vi "Station Initialize.vi"(8 "error in (no error)":errorcluster, 11 "Station in":refnum<class "Station.lvclass">) -> (0 "error out":errorcluster, 2 "All Passed?":bool, 3 "Station out":refnum<class "Station.lvclass">)   [LabVIEW 2018, in "Station.lvclass"]
uses:
  Station.lvclass
  Station Support/Controls/Server Control.ctl
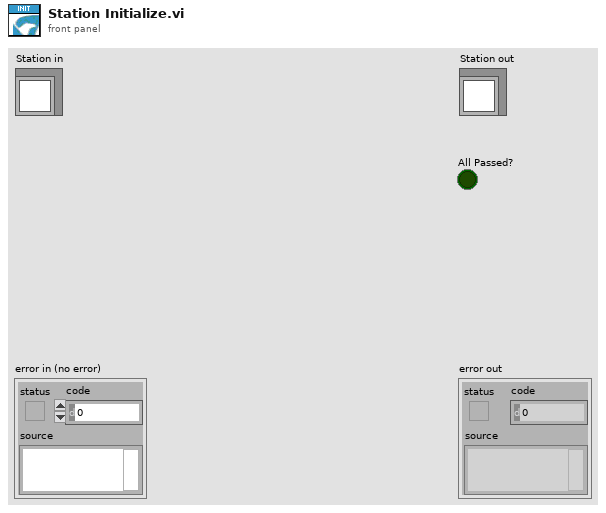
[diagram p1: front panel]
types:
  T1 = typedef "Server Control.ctl" = enum16{"Open New Reference", "Remove Reference", "Kill Server", "Set Station Ref", "Get Station Ref"}
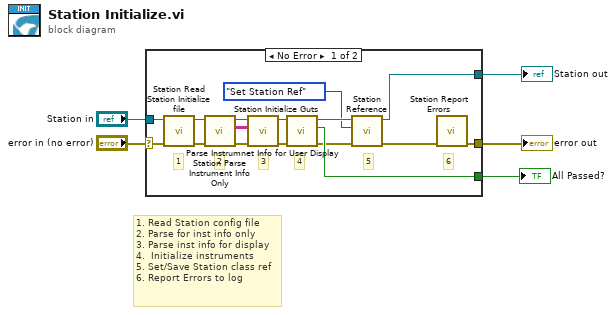
[diagram p0: block diagram]
diagram:
  # "1. Read Station config file\n2. Parse for inst info only\n3. Parse inst info for display\n4.  Initialize instruments\n5. Set/Save Station class ref\n6. Report Errors to log"
  n1 = case shown="No Error" "error in (no error)" {
    selector: "error in (no error)" -> [w21 w23]
    tunnel: [w11 w23] -> w4
    tunnel: [w8 w22] -> w2
    tunnel: "Station in" -> [w20 w22]
    tunnel: [w12 _] -> w1
    frame No Error {
      # "6"
      # "5"
      # "4"
      # "3"
      # "2"
      # "1"
      n2 = call "Station Read Station Initialize file.vi"("error in (no error)"=w21, "Station in"=w20) -> ("error out"=w19:errorcluster, "Station out"=w18:refnum<class "Station.lvclass">)  [unwired: 8 in]
      n3 = call "Station Parse Instrument Info Only.vi"("error in (no error)"=w19, "Station in"=w18) -> ("error out"=w17:errorcluster, "Inst Info only output"=w15:string[][], "Station out"=w16:refnum<class "Station.lvclass">)  [unwired: 7 in]
      n4 = call "Parse Instrumnet Info for User Display.vi"("error in (no error)"=w17, "Inst Info only output"=w15, "Station in"=w16) -> ("error out"=w13:errorcluster, "Station out"=w14:refnum<class "Station.lvclass">)  [unwired: 7 in]
      n5 = call "Station Initialize Guts.vi"("error in (no error)"=w13, "Station in"=w14) -> ("error out"=w10:errorcluster, "All Passed?"=w12:bool, "Station out"=w9:refnum<class "Station.lvclass">)  [unwired: 7 in]
      n6 = call "Station Reference.vi"("error in (no error)"=w10, "Action (0: Create)"=Server_Control."Set Station Ref", "Station in"=w9) -> ("error out"=w7:errorcluster, "Station out"=w8:refnum<class "Station.lvclass">)  [unwired: 7 in]
      n7 = call "Station Report Errors.vi"("error in (no error)"=w7) -> ("error out"=w11:errorcluster)  [unwired: 10 in]
    }
    frame Error {
    }
  }
  "error out" <- w4
  "Station out" <- w2
  "All Passed?" <- w1
